vi "receiver.vi"() -> ()   [LabVIEW 2010]
uses:
  ClassA/ClassA.lvclass
  ClassB/ClassB.lvclass
panel:
  out "number of objects received":i32
  out "type of received objects attribute":string
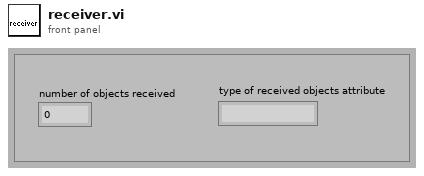
[diagram p1: front panel]
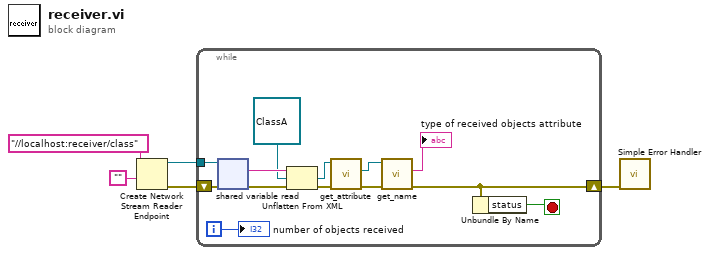
[diagram p0: block diagram]
diagram:
  n1 = Create Network Stream Reader Endpoint(9:"", 11:"//localhost:receiver/class" ("reader url")) -> (0:w5:errorcluster, 3:w3:refnum<k21>)  [unwired: 4 in]
  n2 = while {
    tunnel: w3 -> [w17]
    shift-right: [w9] -> w1
    shift-left: w5 -> [w18]
    i -> [w6]
    stop <- w8 stop-if-true
    n3 = shared-variable-read(w17, w18) -> (w16:errorcluster, w15:string)  [unwired: 1 in, 2 out]
    n4 = Unflatten From XML(xml string=w15, type=refnum<class "ClassA.lvclass"> refnum ("ClassA.lvclass"), error in (no error)=w16) -> (value=w12:refnum<class "ClassA.lvclass">, error out=w13:errorcluster)
    n5 = call "get_attribute.vi"("error in (no error)"=w13, "ClassA in"=w12) -> ("error out"=w11:errorcluster, "ClassB.lvclass"=w10:refnum<class "ClassB.lvclass">)  [unwired: 7 in, 1 out]
    n6 = call-dynamic "get_name.vi"("error in (no error)"=w11, "ClassB in"=w10) -> ("error out"=w9:errorcluster, "name"=→"type of received objects attribute":string)  [unwired: 7 in, 1 out]
    n7 = Unbundle By Name(w9) -> ("status"=w8:bool)
    "number of objects received" <- w6
  }
  n8 = call <vilib>:"Simple Error Handler.vi"("error in (no error)"=w1) -> ()  [unwired: 4 in, 5 out]
